vi "testStringIncluded.vi"() -> (0 "error out":errorcluster)   [LabVIEW 2019, in "AssertionTest.lvlib" / "AssertStringContainsString.lvlib"]
uses:
  AssertStringContainsString.lvlib
  Assertion/Assertion.lvlib
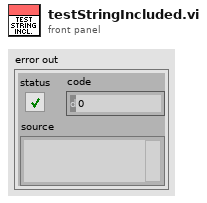
[diagram p1: front panel]
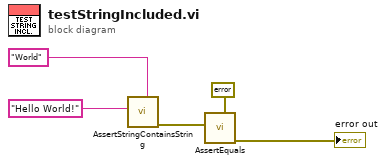
[diagram p0: block diagram]
diagram:
  n1 = call "AssertStringContainsString.vi"("Needle"="World", "Haystack"="Hello World!") -> ("error out"=w3:errorcluster)  [unwired: 9 in]
  n2 = call "AssertEquals.vi"("Expected"=errorcluster {"status"=FALSE, "code"=0, "source"=""} ("error constant"), "Actual"=w3) -> ("error out"=→"error out":errorcluster)  [unwired: 9 in]
